vi "solar_voy_def Quotes Remove.vi"(11 "String":string) -> (3 "String without Comments":string)   [LabVIEW 2018]
doc: "This removes quotes from the string."
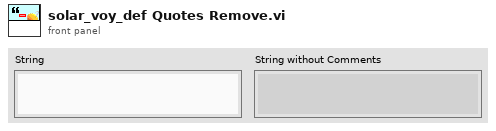
[diagram p1: front panel]
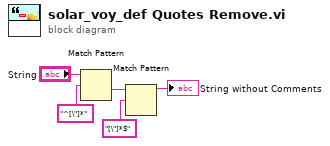
[diagram p0: block diagram]
diagram:
  n1 = Match Pattern(string="String", regular expression="^[\"]*") -> (after substring=w4:string)  [unwired: 1 in, 3 out]
  n2 = Match Pattern(string=w4, regular expression="[\"]*$") -> (before substring=→"String without Comments":string)  [unwired: 1 in, 3 out]
